vi "Measurement Client Utility.vi"(0 "Target Item":refnum<vi>) -> ()   [LabVIEW 2020]
uses:
  <vilib>/gRPC/Generated APIs/ni/measurementlink/discovery/v1/RPC Messages/ni_measurementlink_discovery_v1_EnumerateServicesResponse.ctl
  <vilib>/gRPC/Generated APIs/ni/measurementlink/discovery/v1/RPC Messages/ni_measurementlink_discovery_v1_ServiceDescriptor.ctl
  <vilib>/gRPC/Generated APIs/ni/measurementlink/discovery/v1/RPC Messages/ni_measurementlink_discovery_v1_ServiceDescriptor_AnnotationsEntry.ctl
  <vilib>/gRPC/Generated APIs/ni/measurementlink/discovery/v1/RPC Messages/ni_measurementlink_discovery_v1_EnumerateServicesRequest.ctl
  <vilib>/picture/picture.llb/imagedata.ctl
  <vilib>/gRPC/Generated APIs/ni/measurementlink/discovery/v1/RPC Messages/ni_measurementlink_discovery_v1_ResolveServiceRequest.ctl
  <vilib>/Utility/miscctls.llb/LVPositionTypeDef.ctl
  <vilib>/gRPC/Generated APIs/ni/measurementlink/discovery/v1/ni.measurementlink.discovery.v1.api.lvlib
  <vilib>/Plug-In SDKs/Clients/Discovery V1/NI Discovery V1 Client.lvlib
  <vilib>/Plug-In SDKs/Clients/Measurement Service Client V2/Measurement Service Client V2.lvlib
panel:
  out "Project Name":string
  out "Ctl VIs":refnum<vi>[](array[refnum])
  out "Controls":refnum<vi>[](array[refnum])
  in  "Generate":bool
  out "Output":picture
  out "Configuration":picture
  out "Outputs Descriptor":string
  out "Configs Descriptor":string
  out "service_class":string
  in  "OK":bool
  in  "Available Measurements":string[](tree) caption="Measurement Interface: MyMeasurement (LabVIEW)_LabVIEW"
  out "Target Item Name":string
  out "Enumerate Response":T1
  in  "error in":errorcluster
  out "error out":errorcluster
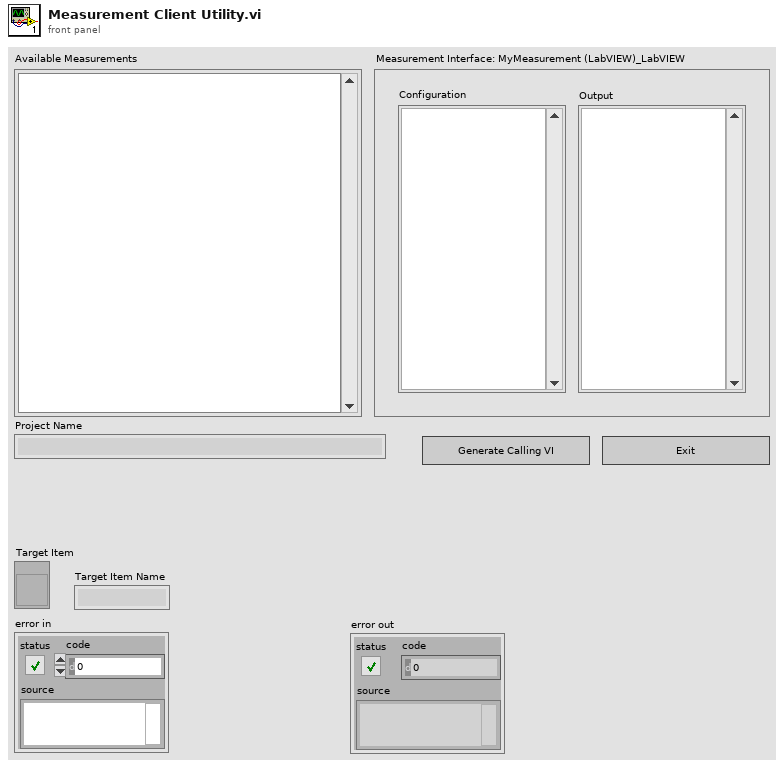
[diagram p1: front panel]
types:
  T1 = typedef "ni.measurementlink.discovery.v1.api.lvlib/ni_measurementlink_discovery_v1_EnumerateServicesResponse.ctl" = cluster{"available_services":T2[]}
  T2 = typedef "ni.measurementlink.discovery.v1.api.lvlib/ni_measurementlink_discovery_v1_ServiceDescriptor.ctl" = cluster{"display_name":string, "description_url":string, "provided_interfaces":string[], "service_class":string, "annotations":T3[]}
  T3 = typedef "ni.measurementlink.discovery.v1.api.lvlib/ni_measurementlink_discovery_v1_ServiceDescriptor_AnnotationsEntry.ctl" = cluster{"key":string, "value":string}
  T4 = typedef "imagedata.ctl" = cluster{"image type":i32, "image depth":i32, "image":u8[], "mask":u8[], "colors":u32[], "Rectangle":cluster{"left":i16, "top":i16, "right":i16, "bottom":i16}}
  T5 = typedef "ni.measurementlink.discovery.v1.api.lvlib/ni_measurementlink_discovery_v1_EnumerateServicesRequest.ctl" = cluster{"provided_interface":string}
  T6 = typedef "ni.measurementlink.discovery.v1.api.lvlib/ni_measurementlink_discovery_v1_ResolveServiceRequest.ctl" = cluster{"provided_interface":string, "service_class":string}
  T7 = typedef "LVPositionTypeDef.ctl" = cluster{"Left":i32, "Top":i32}
  T8 = cluster{"Left Cell String":string, "Child Text":string[], "Child Tag":string, "Item Indent":i32, "Child Only?":bool, "Glyph Index":i32}
  T9 = typedef "grpc-lvsupport-release.lvlib/grpcId.ctl" = u64
  T10 = cluster{"display_name":string, "service_class":string}
  T11 = typedef "ni.measurementlink.discovery.v1.api.lvlib/ni_measurementlink_discovery_v1_ServiceLocation.ctl" = cluster{"location":string, "insecure_port":string, "ssl_authenticated_port":string}
  T12 = typedef "Measurement Service Client V2.lvlib/ni_measurementlink_measurement_v2_GetMetadataResponse.ctl" = cluster{"measurement_details":T13, "measurement_signature":T14, "user_interface_details":T21[]}
  T13 = typedef "Measurement Service Client V2.lvlib/ni_measurementlink_measurement_v2_MeasurementDetails.ctl" = cluster{"display_name":string, "version":string}
  T14 = typedef "Measurement Service Client V2.lvlib/ni_measurementlink_measurement_v2_MeasurementSignature.ctl" = cluster{"configuration_parameters_message_type":string, "configuration_parameters":T15[], "configuration_defaults":T18, "outputs_message_type":string, "outputs":T19[]}
  T15 = typedef "Measurement Service Client V2.lvlib/ni_measurementlink_measurement_v2_ConfigurationParameter.ctl" = cluster{"field_number":i32, "type":T16, "name":string, "repeated":bool, "annotations":T17[], "message_type":string}
  T16 = typedef "Measurement Service Client V2.lvlib/google_protobuf_Field_Kind.ctl" = enum32{"TYPE_UNKNOWN", "TYPE_DOUBLE", "TYPE_FLOAT", "TYPE_INT64", "TYPE_UINT64", "TYPE_INT32", "TYPE_FIXED64", "TYPE_FIXED32", "TYPE_BOOL", "TYPE_STRING", "TYPE_GROUP", "TYPE_MESSAGE", "TYPE_BYTES", "TYPE_UINT32", "TYPE_ENUM", "TYPE_SFIXED32", "TYPE_SFIXED64", "TYPE_SINT32", "TYPE_SINT64"}
  T17 = typedef "Measurement Service Client V2.lvlib/ni_measurementlink_measurement_v2_ConfigurationParameter_AnnotationsEntry.ctl" = cluster{"key":string, "value":string}
  T18 = typedef "Measurement Service Client V2.lvlib/google_protobuf_Any.ctl" = cluster{"type_url":string, "value":u8[]}
  T19 = typedef "Measurement Service Client V2.lvlib/ni_measurementlink_measurement_v2_Output.ctl" = cluster{"field_number":i32, "type":T16, "name":string, "repeated":bool, "annotations":T20[], "message_type":string}
  T20 = typedef "Measurement Service Client V2.lvlib/ni_measurementlink_measurement_v2_Output_AnnotationsEntry.ctl" = cluster{"key":string, "value":string}
  T21 = typedef "Measurement Service Client V2.lvlib/ni_measurementlink_measurement_v2_UserInterfaceDetails.ctl" = cluster{"file_url":string}
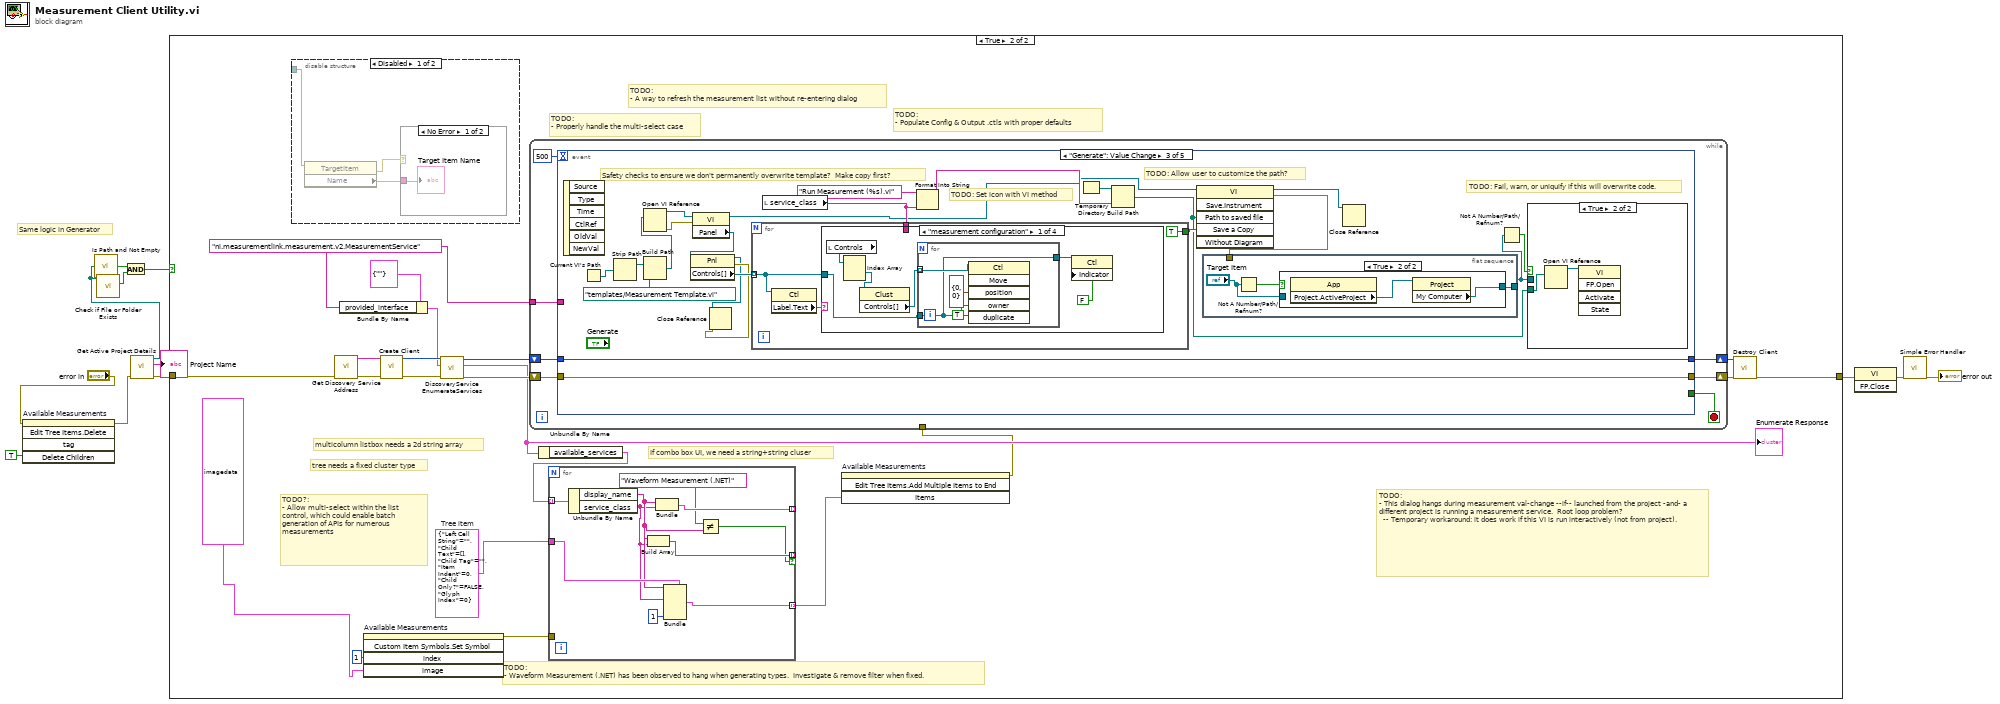
[diagram p0: block diagram]
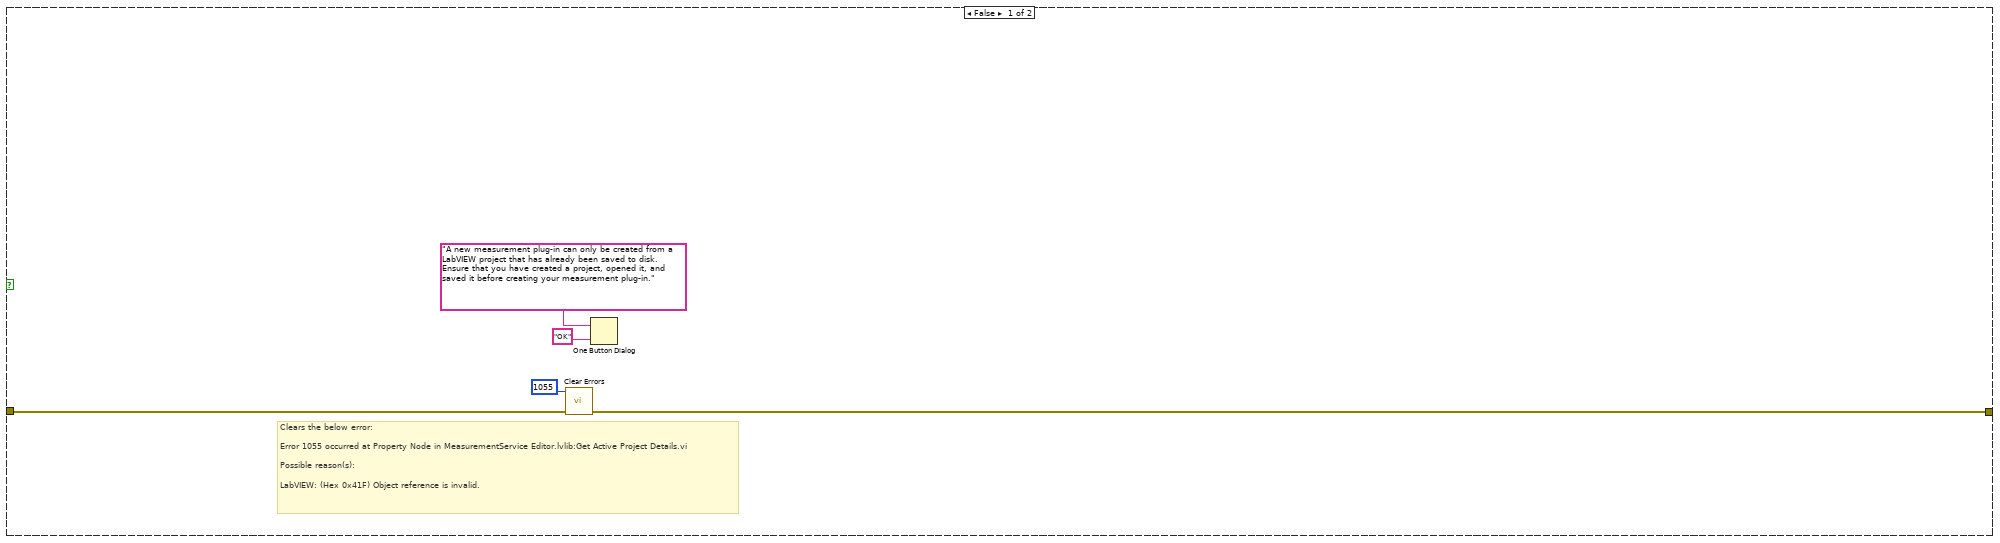
[diagram p2: hidden frame]
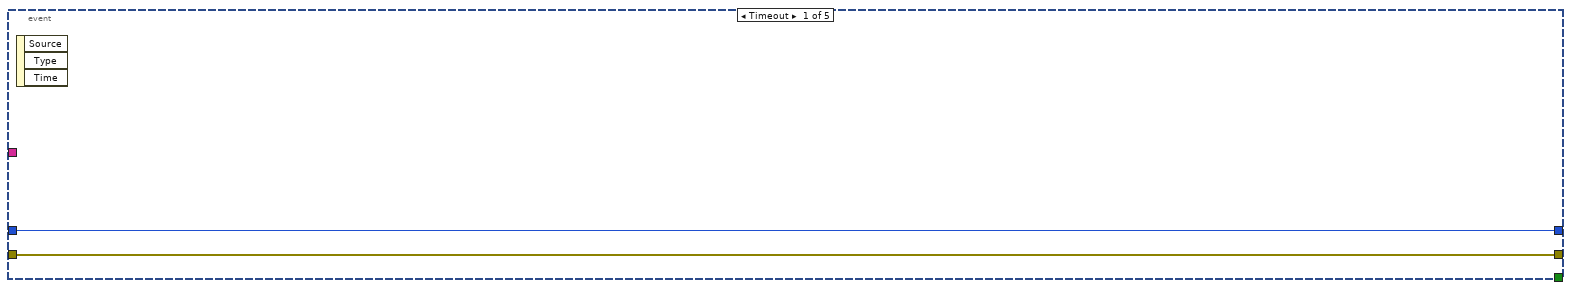
[diagram p5: hidden frame]
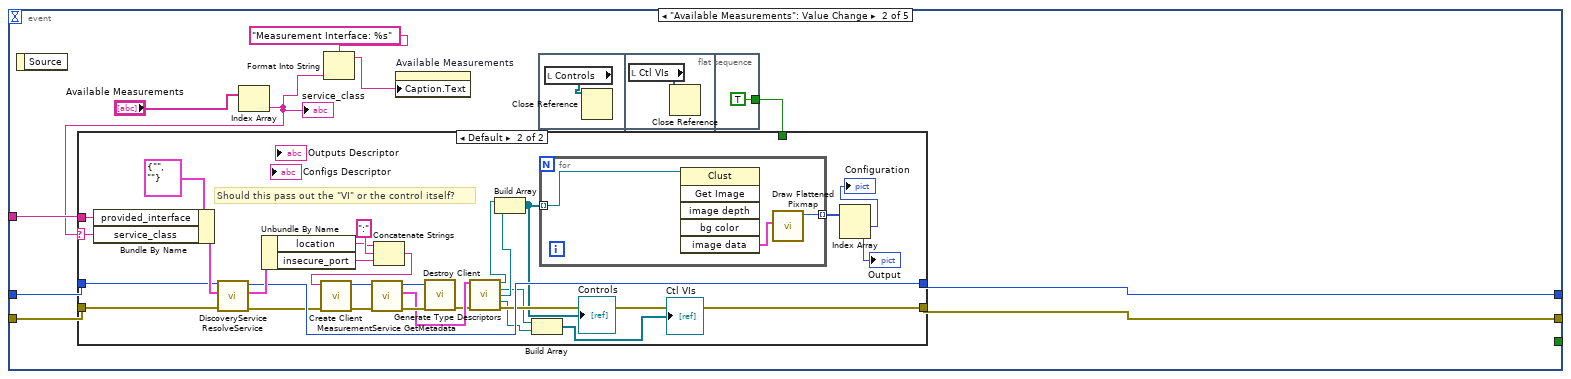
[diagram p6: hidden frame]
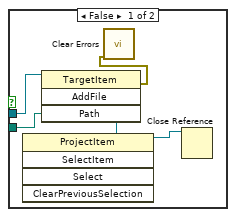
[diagram p8: hidden frame]
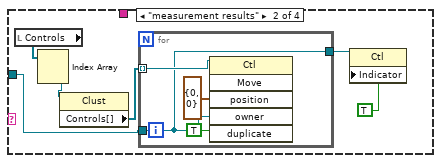
[diagram p10: hidden frame]
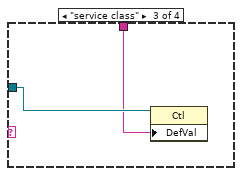
[diagram p11: hidden frame]
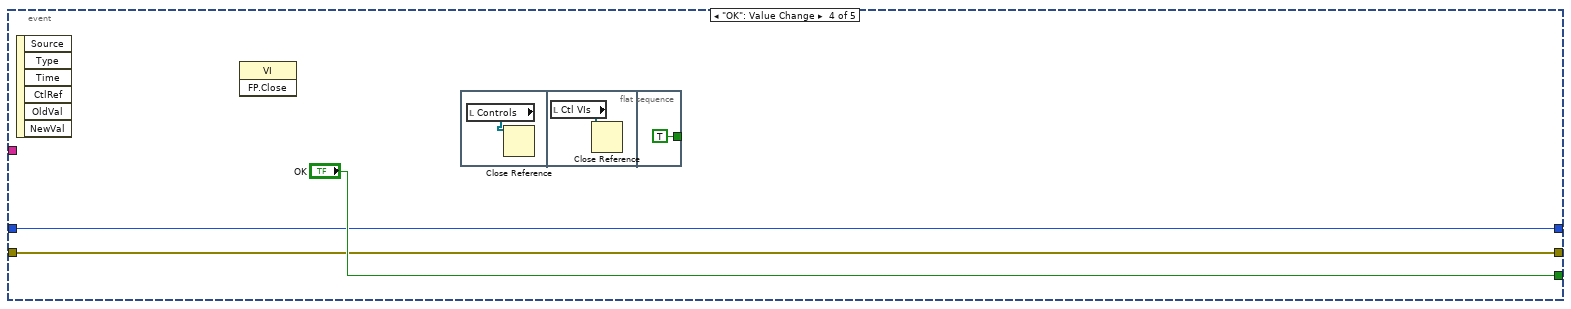
[diagram p13: hidden frame]
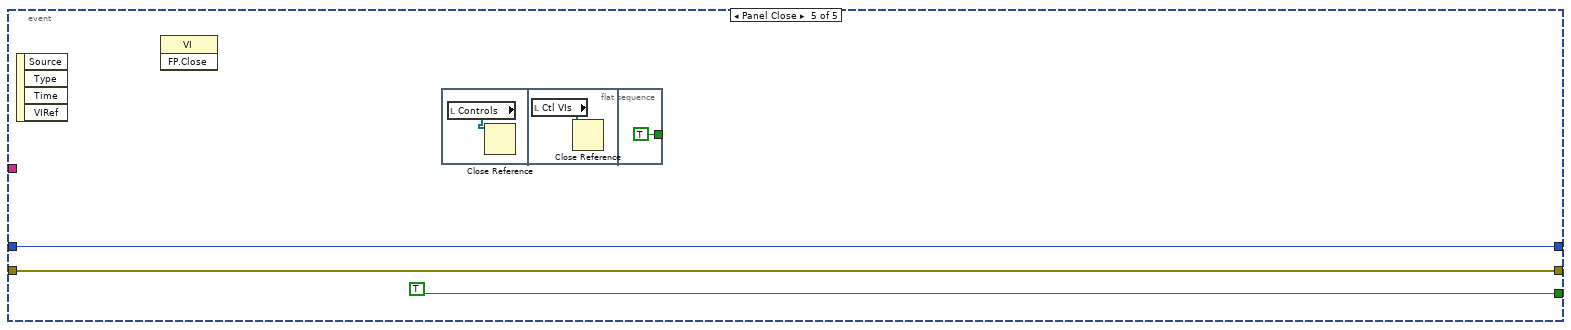
[diagram p14: hidden frame]
diagram:
  # "Same logic in Generator"
  n1 = invoke on="Available Measurements" class="Tree (strict)" method="Edit Tree Items.Delete"(error in="error in", "Delete Children"=TRUE ("Delete Children?")) -> (error out=w1:errorcluster)  [unwired: 3 in, 4 out]
  n2 = call "Get Active Project Details.vi"("error in"=w1) -> ("error out"=w9:errorcluster, "name"=→"Project Name":string, "path"=w6:path)  [unwired: 8 in]
  n3 = call <vilib>:"Is Path and Not Empty.vi"("path"=w6) -> ("Is Path and Not Empty?"=w8:bool)  [unwired: 4 in]
  n4 = call <vilib>:"Check if File or Folder Exists.vi"("path"=w6) -> ("file or folder exists?"=w7:bool)  [unwired: 8 in, 2 out]
  n5 = And(x=w8, y=w7) -> (x .and. y?=w5:bool)
  n6 = case shown="True" w5 {
    tunnel: [w14 w25] -> w11
    tunnel: w9 -> [w13 w24]
    frame False {
      # "Clears the below error:\n\nError 1055 occurred at Property Node in MeasurementService Editor.lvlib:Get Active Project Details.vi\n\nPossible reason(s):\n\nLabVIEW: (Hex 0x41F) Object reference is invalid."
      n7 = call <vilib>:"Clear Errors.vi"("error in (no error)"=w13, "specific error code to clear (0: all)"=1055) -> ("error out"=w14:errorcluster)  [unwired: 4 in, 1 out]
      n8 = One Button Dialog(message="A new measurement plug-in can only be created from a LabVIEW project that has already been saved to disk.  Ensure that you have created a project, opened it, and saved it before creating your measurement plug-in.", button name ("OK")="OK") -> ()  [unwired: 1 out]
    }
    frame True {
      w23 = T8 {"Left Cell String"="", "Child Text"=[], "Child Tag"="", "Item Indent"=0, "Child Only?"=FALSE, "Glyph Index"=0}  # Tree item
      w28 = "ni.measurementlink.measurement.v2.MeasurementService" ("provided_interface")
      # "TODO: \n- Properly handle the multi-select case"
      # "tree needs a fixed cluster type"
      # "multicolumn listbox needs a 2d string array"
      # "TODO?: \n- Allow multi-select within the list control, which could enable batch generation of APIs for numerous measurements"
      # "TODO: \n- Populate Config & Output .ctls with proper defaults"
      # "TODO: \n- This dialog hangs during measurement val-change --if-- launched from the project -and- a different project is running a measurement service.  Root loop problem?\n  -- Temporary workaround: it does work if this VI is run interactively (not from project)."
      # "TODO: \n- Waveform Measurement (.NET) has been observed to hang when generating types.  Investigate & remove filter when fixed."
      # "If combo box UI, we need a string+string cluser"
      # "TODO: \n- A way to refresh the measurement list without re-entering dialog"
      n9 = disable-structure shown="Disabled" {
        disable-tunnel: _ -> [w41 _]
        frame Disabled {
          n10 = property class="TargetItem"(reference=w41) -> (error out=w39:errorcluster, "Name"=w40:string)  [unwired: 1 in, 1 out]
          n11 = case shown="No Error" w39 {
            tunnel: w40 -> [w42 _]
            frame No Error {
              "Target Item Name" <- w42
            }
            frame Error {
            }
          }
        }
        frame Enabled {
        }
      }
      n12 = call <vilib>:"Get Discovery Service Address.vi"("error in"=w24) -> ("error out"=w32:errorcluster, "address"=w31:string)  [unwired: 9 in]
      n13 = Bundle By Name(cluster=T5 {"provided_interface"=""} ("Request Data"), "provided_interface"=w28) -> (w29:T5)
      n14 = invoke on="Available Measurements" class="Tree (strict)" method="Custom Item Symbols.Set Symbol"("index"=1 ("Index"), "image"=T4 {"image type"=0, "image depth"=24, "image"=[255, 255, 255, 255, 255, 255, 255, 255, 255, 255, 255, 255, 255, 255, 255, 255, 255, 255, 255, 255, 255, 255, 255, 255, 255, 255, 255, 255, 255, 255, 255, 255, 255, 255, 255, 255, 255, 255, 255, 255, 255, 255, 255, 255, 255, 255, 255, 255, 255, 255, 255, 255, 255, 255, 255, 255, 255, 255, 255, 255, 255, 255, 255, 255, 255, 255, 255, 255, 255, 255, 255, 255, 255, 255, 255, 255, 255, 255, 255, 255, 255, 255, 255, 255, 255, 255, 255, 255, 255, 255, 255, 255, 255, 255, 255, 255, 255, 255, 255, 255, 255, 255, 255, 255, 255, 255, 255, 255, 255, 255, 255, 255, 255, 255, 255, 255, 255, 12, 12, 12, 12, 12, 12, 255, 255, 255, 255, 255, 255, 255, 255, 255, 255, 255, 255, 255, 255, 255, 255, 255, 255, 255, 255, 255, 255, 255, 255, 255, 255, 255, 255, 255, 255, 255, 255, 255, 255, 255, 255, 255, 255, 255, 255, 255, 255, 0, 0, 0, 0, 0, 0, 255, 255, 255, 255, 255, 255, 255, 255, 255, 255, 255, 255, 255, 255, 255, 255, 255, 255, 255, 255, 255, 255, 255, 255, 255, 255, 255, 255, 255, 255, 255, 255, 255, 255, 255, 255, 255, 255, 255, 82, 82, 82, 0, 0, 0, 0, 0, 0, 74, 74, 74, 255, 255, 255, 255, 255, 255, 255, 255, 255, 255, 255, 255, 255, 255, 255, 255, 255, 255, 255, 255, 255, 255, 255, 255, 255, 255, 255, 255, 255, 255, 255, 255, 255, 118, 118, 118, 108, 108, 108, 254, 254, 254, 254, 254, 254, 108, 108, 108, 116, 116, 116, 255, 255, 255, 255, 255, 255, 255, 255, 255, 255, 255, 255, 255, 255, 255, 255, 255, 255, 255, 255, 255, 255, 255, 255, 255, 255, 255, 181, 181, 181, 120, 120, 120, 196, 196, 196, 181, 181, 181, 181, 181, 181, 196, 196, 196, 120, 120, 120, 178, 178, 178, 255, 255, 255, 255, 255, 255, 255, 255, 255, 255, 255, 255, 255, 255, 255, 255, 255, 255, 255, 255, 255, 255, 255, 255, 157, 157, 157, 184, 184, 184, 255, 255, 255, 0, 0, 0, 0, 0, 0, 255, 255, 255, 184, 184, 184, 152, 152, 152, 255, 255, 255, 255, 255, 255, 255, 255, 255, 255, 255, 255, 255, 255, 255, 255, 255, 255, 255, 255, 255, 255, 255, 255, 152, 152, 152, 162, 162, 162, 236, 236, 236, 34, 34, 34, 34, 34, 34, 236, 236, 236, 162, 162, 162, 150, 150, 150, 255, 255, 255, 255, 255, 255, 255, 255, 255, 255, 255, 255, 255, 255, 255, 255, 255, 255, 255, 255, 255, 255, 255, 255, 105, 105, 105, 28, 28, 28, 130, 130, 130, 255, 255, 255, 255, 255, 255, 130, 130, 130, 28, 28, 28, 106, 106, 106, 255, 255, 255, 255, 255, 255, 255, 255, 255, 255, 255, 255, 255, 255, 255, 255, 255, 255, 255, 255, 255, 166, 166, 166, 38, 38, 38, 20, 20, 20, 58, 58, 58, 102, 102, 102, 102, 102, 102, 58, 58, 58, 20, 20, 20, 38, 38, 38, 168, 168, 168, 255, 255, 255, 255, 255, 255, 255, 255, 255, 255, 255, 255, 255, 255, 255, 255, 255, 255, 58, 58, 58, 24, 24, 24, 151, 151, 151, 255, 255, 255, 226, 226, 226, 226, 226, 226, 255, 255, 255, 151, 151, 151, 24, 24, 24, 60, 60, 60, 255, 255, 255, 255, 255, 255, 255, 255, 255, 255, 255, 255, 255, 255, 255, 188, 188, 188, 22, 22, 22, 116, 116, 116, 255, 255, 255, 255, 255, 255, 255, 255, 255, 255, 255, 255, 255, 255, 255, 255, 255, 255, 116, 116, 116, 24, 24, 24, 204, 204, 204, 255, 255, 255, 255, 255, 255, 255, 255, 255, 255, 255, 255, 38, 38, 38, 54, 54, 54, 255, 255, 255, 255, 255, 255, 103, 103, 103, 51, 51, 51, 51, 51, 51, 103, 104, 104, 255, 255, 255, 255, 255, 255, 54, 54, 54, 42, 42, 42, 255, 255, 255, 255, 255, 255, 255, 255, 255, 228, 228, 228, 144, 144, 144, 255, 255, 255, 255, 255, 255, 255, 255, 255, 255, 255, 255, 255, 255, 255, 255, 255, 255, 255, 255, 255, 255, 255, 255, 255, 255, 255, 255, 255, 255, 140, 140, 140, 240, 240, 240, 255, 255, 255, 255, 255, 255, 255, 255, 255, 255, 255, 255, 255, 255, 255, 255, 255, 255, 255, 255, 255, 255, 255, 255, 255, 255, 255, 255, 255, 255, 255, 255, 255, 255, 255, 255, 255, 255, 255, 255, 255, 255, 255, 255, 255, 255, 255, 255, 255, 255, 255], "mask"=[], "colors"=[], "Rectangle"={"left"=0, "top"=0, "right"=16, "bottom"=16}} ("image data")) -> (error out=w19:errorcluster)  [unwired: 3 in, 4 out]
      n15 = call <vilib>:"Create Client.vi"("error in"=w32, "address"=w31) -> ("error out"=w34:errorcluster, "gRPC ID Out"=w33:T9)  [unwired: 8 in]
      n16 = call <vilib>:"DiscoveryService EnumerateServices.vi"("error in"=w34, "Request Data"=w29, "gRPC ID"=w33) -> ("error out"=w36:errorcluster, "Response Data"=w27:T1, "gRPC ID out"=w35:T9)  [unwired: 6 in]
      "Enumerate Response" <- w27
      n17 = Unbundle By Name(w27) -> ("available_services"=w26:T2[])
      n18 = for {
        tunnel: w26 -> [w182] mode=indexing
        tunnel: [w181] -> _ mode=indexing
        tunnel: [w180] -> _ mode=indexing if=w178
        tunnel: w23 -> [w177]
        tunnel: [w174] -> w22 mode=indexing
        tunnel: w19 -> [_]
        n19 = Unbundle By Name(w182) -> ("display_name"=w176:string, "service_class"=w175:string)
        n20 = Build Array(w176, w175) -> (w180:string[])
        n21 = Bundle("display_name"=w176, "service_class"=w175) -> (w181:T10)  [unwired: 1 in]
        n22 = Bundle(cluster=w177, "Left Cell String"=w176, "Child Tag"=w175, "Glyph Index"=1) -> (w174:T8)  [unwired: 3 in]
        n23 = Not Equal?(x="Waveform Measurement (.NET)", y=w176) -> (x != y?=w178:bool)
      }
      n24 = invoke on="Available Measurements" class="Tree (strict)" method="Edit Tree Items.Add Multiple Items to End"("Items"=w22) -> (error out=w21:errorcluster)  [unwired: 3 in, 3 out]
      n25 = while {
        shift-right: [w48] -> w37
        shift-left: w36 -> [w47]
        shift-right: [w49] -> w38
        shift-left: w35 -> [w46]
        tunnel: w28 -> [w45]
        tunnel: w21 -> [_]
        stop <- w44 stop-if-true
        n26 = event shown="[2] \"Generate\": Value Change" {
          selector: _ -> [_ _ _ _ _]
          dyn-events: _ -> [_ _ _ _ _]
          timeout: 500 -> [_ _ _ _ _]
          tunnel: [w51 w61 w121 w161 w168] -> w49
          tunnel: [w50 w60 w120 w162 w169] -> w48
          tunnel: w47 -> [w50 w59 w120 w162 w169]
          tunnel: w46 -> [w51 w58 w121 w161 w168]
          tunnel: w45 -> [_ w57 _ _ _]
          tunnel: [_ _ _ "OK" TRUE ("OK")] -> w44
          event Timeout {
            n27 = event-data() -> ()  [unwired: 1 in, 3 out]
          }
          event "Available Measurements": Value Change {
            n28 = event-data() -> ()  [unwired: 1 in, 1 out]
            n29 = Index Array(array="Available Measurements") -> (element=w53:string)  [unwired: 1 in]
            "service_class" <- w53
            n30 = case shown="Default" w53 {
              selector: w53 -> [_ w79]
              tunnel: [w65 w89] -> w61
              tunnel: [w66 w77] -> w60
              tunnel: w59 -> [w66 w88]
              tunnel: w58 -> [w65 w87]
              tunnel: w57 -> [_ w86]
              tunnel: w56 -> [_ _]
              frame "" {
              }
              frame Default {
                # "Should this pass out the \"VI\" or the control itself?"
                n31 = Bundle By Name(cluster=T6 {"provided_interface"="", "service_class"=""} ("Request Data"), "provided_interface"=w86, "service_class"=w79) -> (w91:T6)
                n32 = call <vilib>:"DiscoveryService ResolveService.vi"("error in"=w88, "Request Data"=w91, "gRPC ID"=w87) -> ("error out"=w80:errorcluster, "Response Data"=w92:T11, "gRPC ID out"=w89:T9)  [unwired: 6 in]
                n33 = Unbundle By Name(w92) -> ("location"=w93:string, "insecure_port"=w95:string)
                n34 = Concatenate Strings(w93, ":" ("string"), w95) -> (w81:string)
                n35 = call <vilib>:"Create Client.vi"("error in"=w80, "address"=w81) -> ("error out"=w82:errorcluster, "gRPC ID Out"=w83:T9)  [unwired: 8 in]
                n36 = call <vilib>:"MeasurementService GetMetadata.vi"("error in"=w82, "gRPC ID"=w83) -> ("error out"=w84:errorcluster, "Response Data"=w78:T12, "gRPC ID out"=w85:T9)  [unwired: 7 in]
                n37 = call <vilib>:"Destroy Client.vi"("error in"=w84, "gRPC ID"=w85) -> ("error out"=w76:errorcluster)  [unwired: 9 in]
                n38 = call "Generate Type Descriptors.vi"("Measurement Metadata"=w78, "error in (no error)"=w76) -> ("Configs Type"=w75:refnum<vi>, "Configs Ctl"=w69:refnum<vi>, "Outputs Type"=w74:refnum<vi>, "Outputs Ctl"=w68:refnum<vi>, "error out"=w77:errorcluster)  [unwired: 9 in]
                n39 = Build Array(w75, w74) -> (w73:refnum<vi>[])
                "Controls" <- w73
                n40 = Build Array(w69, w68) -> (→"Ctl VIs":refnum<vi>[])
                n41 = for {
                  tunnel: w73 -> [w96] mode=indexing
                  tunnel: [w97] -> w72 mode=indexing
                  n42 = invoke class="Clust" method="Get Image"(reference=w96) -> ("image data"=w98:T4)  [unwired: 5 in, 5 out]
                  n43 = call <vilib>:"Draw Flattened Pixmap.vi"("image data"=w98) -> ("new picture"=w97:picture)  [unwired: 8 in]
                }
                n44 = Index Array(array=w72) -> (element #1=→"Configuration":picture, element #2=→"Output":picture)  [unwired: 2 in]
              }
            }
            n45 = Format Into String(format string="Measurement Interface: %s", w53) -> (resulting string=w54:string)  [unwired: 2 in, 1 out]
            n46 = property on="Available Measurements" class="Tree (strict)"("Caption.Text"=w54) -> ()  [unwired: 2 in, 2 out]
            n47 = flat-sequence {
              tunnel: [TRUE] -> w56
              frame #0 {
                n48 = local read "Controls"() -> (w62:refnum<vi>[])
                n49 = Close Reference(reference=w62) -> ()  [unwired: 1 in, 1 out]
              }
              frame #1 {
                n50 = local read "Ctl VIs"() -> (w63:refnum<vi>[])
                n51 = Close Reference(reference=w63) -> ()  [unwired: 1 in, 1 out]
              }
              frame #2 {
              }
            }
          }
          event "Generate": Value Change {
            # "TODO: Allow user to customize the path?"
            # "TODO: Fail, warn, or uniquify if this will overwrite code."
            # "TODO: Set icon with VI method"
            # "Safety checks to ensure we don't permanently overwrite template?  Make copy first?"
            n52 = event-data() -> ()  [unwired: 1 in, 6 out]
            n53 = Current VI's Path() -> (path=w117:path)
            n54 = Strip Path(path=w117) -> (stripped path=w119:path)  [unwired: 1 out]
            n55 = Build Path(base path=w119, name or relative path=path "templates/Measurement Template.vi") -> (appended path=w116:path)
            n56 = Open VI Reference(vi path=w116) -> (vi reference=w114:refnum<vi>, error out=w115:errorcluster)  [unwired: 5 in]
            n57 = property class="VI"(reference=w114, error in=w115) -> (reference out=w101:refnum<vi>, "Panel"=w113:refnum<vi>)  [unwired: 1 out]
            n58 = property class="Pnl"(reference=w113) -> (reference out=w104:refnum<vi>, error out=w105:errorcluster, "Controls[]"=w112:refnum<vi>[])  [unwired: 1 in]
            n59 = Close Reference(reference=w104, error in (no error)=w105) -> ()  [unwired: 1 out]
            n60 = local read "service_class"() -> (w110:string)
            n61 = for {
              tunnel: w112 -> [w137] mode=indexing
              tunnel: w110 -> [w136]
              tunnel: [TRUE] -> w107
              n62 = property class="Ctl"(reference=w137) -> ("Label.Text"=w138:string)  [unwired: 1 in, 2 out]
              n63 = case shown="\"measurement configuration\"" w138 {
                tunnel: w137 -> [w142 w151 w160 _]
                tunnel: w136 -> [_ _ w159 _]
                frame "measurement configuration" {
                  n64 = local read "Controls"() -> (w144:refnum<vi>[])
                  n65 = Index Array(array=w144) -> (element #1=w139:refnum<vi>)  [unwired: 2 in, 1 out]
                  n66 = property class="Clust"(reference=w139) -> ("Controls[]"=w143:refnum<vi>[])  [unwired: 1 in, 2 out]
                  n67 = for {
                    tunnel: w143 -> [w148] mode=indexing
                    tunnel: w142 -> [w145]
                    tunnel: [w145] -> w141
                    n68 = invoke class="Ctl" method="Move"(reference=w148, "position"=T7 {"Left"=0, "Top"=0}, "owner"=w145, "duplicate"=TRUE ("Duplicate? (F)")) -> ()  [unwired: 2 in, 6 out]
                  }
                  n69 = property class="Ctl"(reference=w141, "Indicator"=FALSE) -> ()  [unwired: 1 in, 2 out]
                }
                frame "measurement results" {
                  n70 = local read "Controls"() -> (w154:refnum<vi>[])
                  n71 = Index Array(array=w154) -> (element #2=w153:refnum<vi>)  [unwired: 2 in, 1 out]
                  n72 = property class="Clust"(reference=w153) -> ("Controls[]"=w152:refnum<vi>[])  [unwired: 1 in, 2 out]
                  n73 = for {
                    tunnel: w152 -> [w158] mode=indexing
                    tunnel: w151 -> [w155]
                    tunnel: [w155] -> w150
                    n74 = invoke class="Ctl" method="Move"(reference=w158, "position"=T7 {"Left"=0, "Top"=0}, "owner"=w155, "duplicate"=TRUE ("Duplicate? (F)")) -> ()  [unwired: 2 in, 6 out]
                  }
                  n75 = property class="Ctl"(reference=w150, "Indicator"=TRUE) -> ()  [unwired: 1 in, 2 out]
                }
                frame "service class" {
                  n76 = property class="Ctl"(reference=w160, "DefVal"=w159) -> ()  [unwired: 1 in, 2 out]
                }
                frame Default {
                }
              }
            }
            n77 = Format Into String(format string="Run Measurement (%s).vi", w110) -> (resulting string=w108:string)  [unwired: 2 in, 1 out]
            n78 = Temporary Directory() -> (w109:path)
            n79 = Build Path(base path=w109, name or relative path=w108) -> (appended path=w102:path)
            n80 = invoke class="VI" method="Save.Instrument"(reference=w101, "Path to saved file"=w102, "Save a Copy"=w107) -> (reference out=w106:refnum<vi>, error out=w103:errorcluster)  [unwired: 3 in, 4 out]
            n81 = flat-sequence {
              tunnel: [w130] -> w100
              tunnel: w103 -> [_]
              frame #0 {
                n82 = Not A Number/Path/Refnum?(number/path/refnum="Target Item") -> (NaN/Path/Refnum?=w131:bool)
                n83 = case shown="True" w131 {
                  tunnel: [w132 w133] -> w130
                  tunnel: "Target Item" -> [w132 _]
                  frame False {
                  }
                  frame True {
                    n84 = property class="App"() -> ("Project.ActiveProject"=w134:refnum<vi>)  [unwired: 2 in, 2 out]
                    n85 = property class="Project"(reference=w134) -> ("My Computer"=w133:refnum<vi>)  [unwired: 1 in, 2 out]
                  }
                }
              }
            }
            n86 = Close Reference(reference=w106) -> ()  [unwired: 1 in, 1 out]
            n87 = Not A Number/Path/Refnum?(number/path/refnum=w100) -> (NaN/Path/Refnum?=w99:bool)
            n88 = case shown="True" w99 {
              tunnel: w102 -> [w124 w128]
              tunnel: w100 -> [w126 _]
              frame False {
                n89 = invoke class="TargetItem" method="AddFile"(reference=w126, "Path"=w124) -> (error out=w125:errorcluster, "AddFile"=w123:refnum<vi>)  [unwired: 2 in, 2 out]
                n90 = invoke class="ProjectItem" method="SelectItem"(reference=w123) -> (reference out=w122:refnum<vi>)  [unwired: 4 in, 4 out]
                n91 = call <vilib>:"Clear Errors.vi"("error in (no error)"=w125) -> ()  [unwired: 5 in, 2 out]
                n92 = Close Reference(reference=w122) -> ()  [unwired: 1 in, 1 out]
              }
              frame True {
                n93 = Open VI Reference(vi path=w128) -> (vi reference=w127:refnum<vi>)  [unwired: 5 in, 1 out]
                n94 = invoke class="VI" method="FP.Open"(reference=w127) -> ()  [unwired: 4 in, 5 out]
              }
            }
          }
          event "OK": Value Change {
            n95 = event-data() -> ()  [unwired: 1 in, 6 out]
            n96 = invoke class="VI" method="FP.Close"() -> ()  [unwired: 3 in, 3 out]
            n97 = flat-sequence {
              tunnel: [TRUE] -> _
              frame #0 {
                n98 = local read "Controls"() -> (w164:refnum<vi>[])
                n99 = Close Reference(reference=w164) -> ()  [unwired: 1 in, 1 out]
              }
              frame #1 {
                n100 = local read "Ctl VIs"() -> (w165:refnum<vi>[])
                n101 = Close Reference(reference=w165) -> ()  [unwired: 1 in, 1 out]
              }
              frame #2 {
              }
            }
          }
          event Panel Close {
            n102 = event-data() -> ()  [unwired: 1 in, 4 out]
            n103 = invoke class="VI" method="FP.Close"() -> ()  [unwired: 3 in, 3 out]
            n104 = flat-sequence {
              tunnel: [TRUE] -> _
              frame #0 {
                n105 = local read "Controls"() -> (w170:refnum<vi>[])
                n106 = Close Reference(reference=w170) -> ()  [unwired: 1 in, 1 out]
              }
              frame #1 {
                n107 = local read "Ctl VIs"() -> (w171:refnum<vi>[])
                n108 = Close Reference(reference=w171) -> ()  [unwired: 1 in, 1 out]
              }
              frame #2 {
              }
            }
          }
        }
      }
      n109 = call <vilib>:"Destroy Client.vi"("error in"=w37, "gRPC ID"=w38) -> ("error out"=w25:errorcluster)  [unwired: 9 in]
    }
  }
  n110 = invoke class="VI" method="FP.Close"(error in=w11) -> (error out=w12:errorcluster)  [unwired: 2 in, 2 out]
  n111 = call <vilib>:"Simple Error Handler.vi"("error in (no error)"=w12) -> ("error out"=→"error out":errorcluster)  [unwired: 4 in, 4 out]
